vi "QuadRotor_Monitoring_LV4.vi"() -> ()   [LabVIEW 2015]
uses:
  <vilib>/Instr/_visa.llb/VISA Set IO Buffer Mask.ctl
  <vilib>/Instr/_visa.llb/VISA Configure Serial Port (Instr).vi
panel:
  out "GPS_TRANSPORT_Distance":dbl(slide) scale=0.0..200.0
  out "GPS_Home_Distance":dbl(slide) scale=0.0..200.0
  out "GPS_Speed_Gaud":ext(knob) scale=0.0..100.0
  out "GPS_LON_TRANSPORT":ext format="%#.7f"
  out "GPS_LAT_TRANSPORT":ext format="%#.7f"
  out "GPS_LON_HOME":ext format="%#.7f"
  out "GPS_LAT_HOME":ext format="%#.7f"
  out "MotorBackRf":dbl(slide) scale=1000.0..2000.0
  out "MotorBackLf":dbl(slide) scale=1000.0..2000.0
  out "MotorFrontRf":dbl(slide) scale=1000.0..2000.0
  out "MotorFrontLf":dbl(slide) scale=1000.0..2000.0
  in  "LON_TRANSPORT":i32=1001113510
  in  "LAT_TRANSPORT":i32=200300620
  in  "LON_HOME":i32=1001110710
  in  "LAT_HOME":i32=200292880
  out "(GPS_numSat)":u16(slide) scale=0.0..20.0 scale format="%#_4g"
  out "return count 2":u32
  out "Roob":i32
  out "Altitude_(Auto)":ext format="%#_3g"
  in  "Set_ATL_(Auto)":dbl=12.0
  out "string":string
  out "Mode":ext format="%.2f"
  out "Altitude":dbl(slide) scale=0.0..20.0
  out "Altitude":ext format="%.2f"
  out "Yaw":dbl(knob) scale=-180.0..180.0
  out "Pitch":dbl(knob) scale=-90.0..90.0
  out "Roll":dbl(knob) scale=-90.0..90.0
  in  "Write to Quad":bool
  out "Header_58":u8
  out "GPS_LONGTITUDE":ext format="%#.7f"
  out "GPS_LATTITUDE":ext format="%#.7f"
  out "return count":u32
  in  "stop":bool
  in  "VISA Serial Data":refnum<visa-resource-name>
  # "Quad Rotor Monitoring and Control with GPS Waypoint"
  # "Data Write to Autonomous Quad Rotor (LAT 9 Point), (LON 10 Point) with Google Map tracking Navigator"
  # "Ex  13.8591411 = 138591411 , 100.5231704 = 1005231704 Using in integer  I32"
  # "GPS Status and Monitoring"
  # "Km/h"
  # "9 Point"
  # "10 Point"
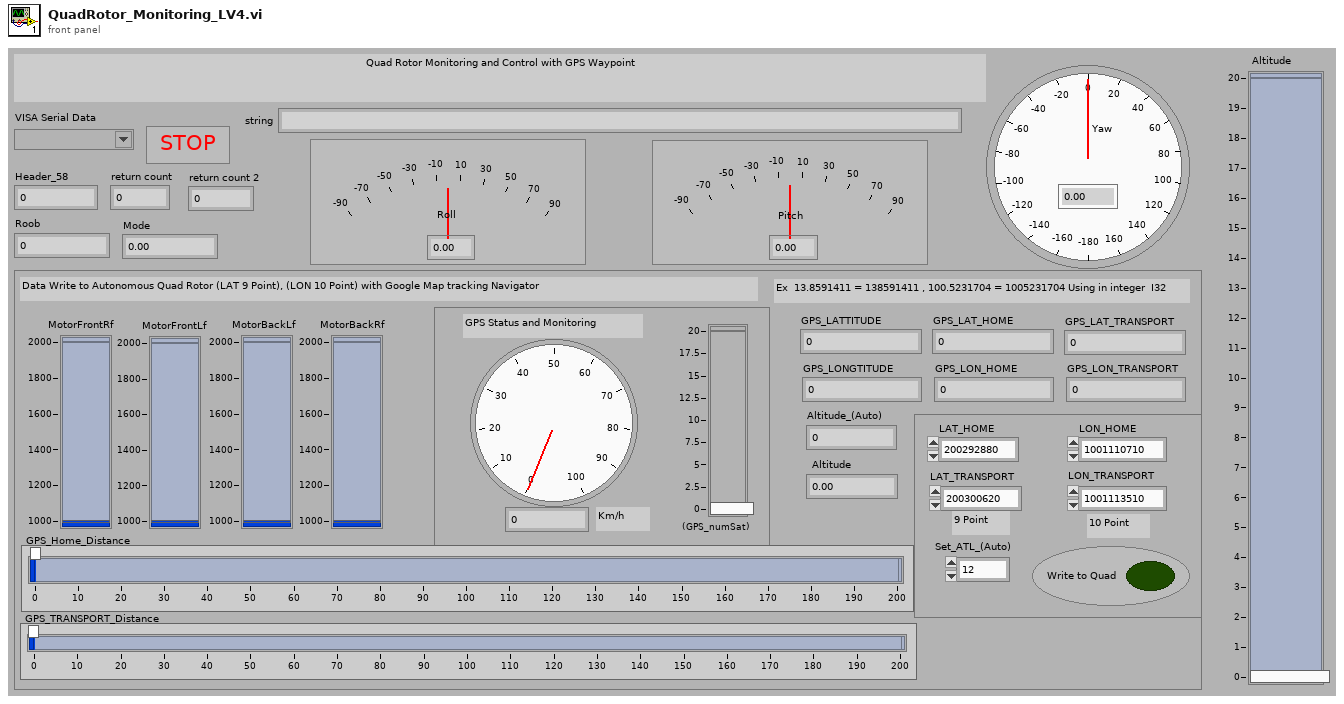
[diagram p1: front panel]
types:
  T1 = typedef "VISA Set IO Buffer Mask.ctl" = u16
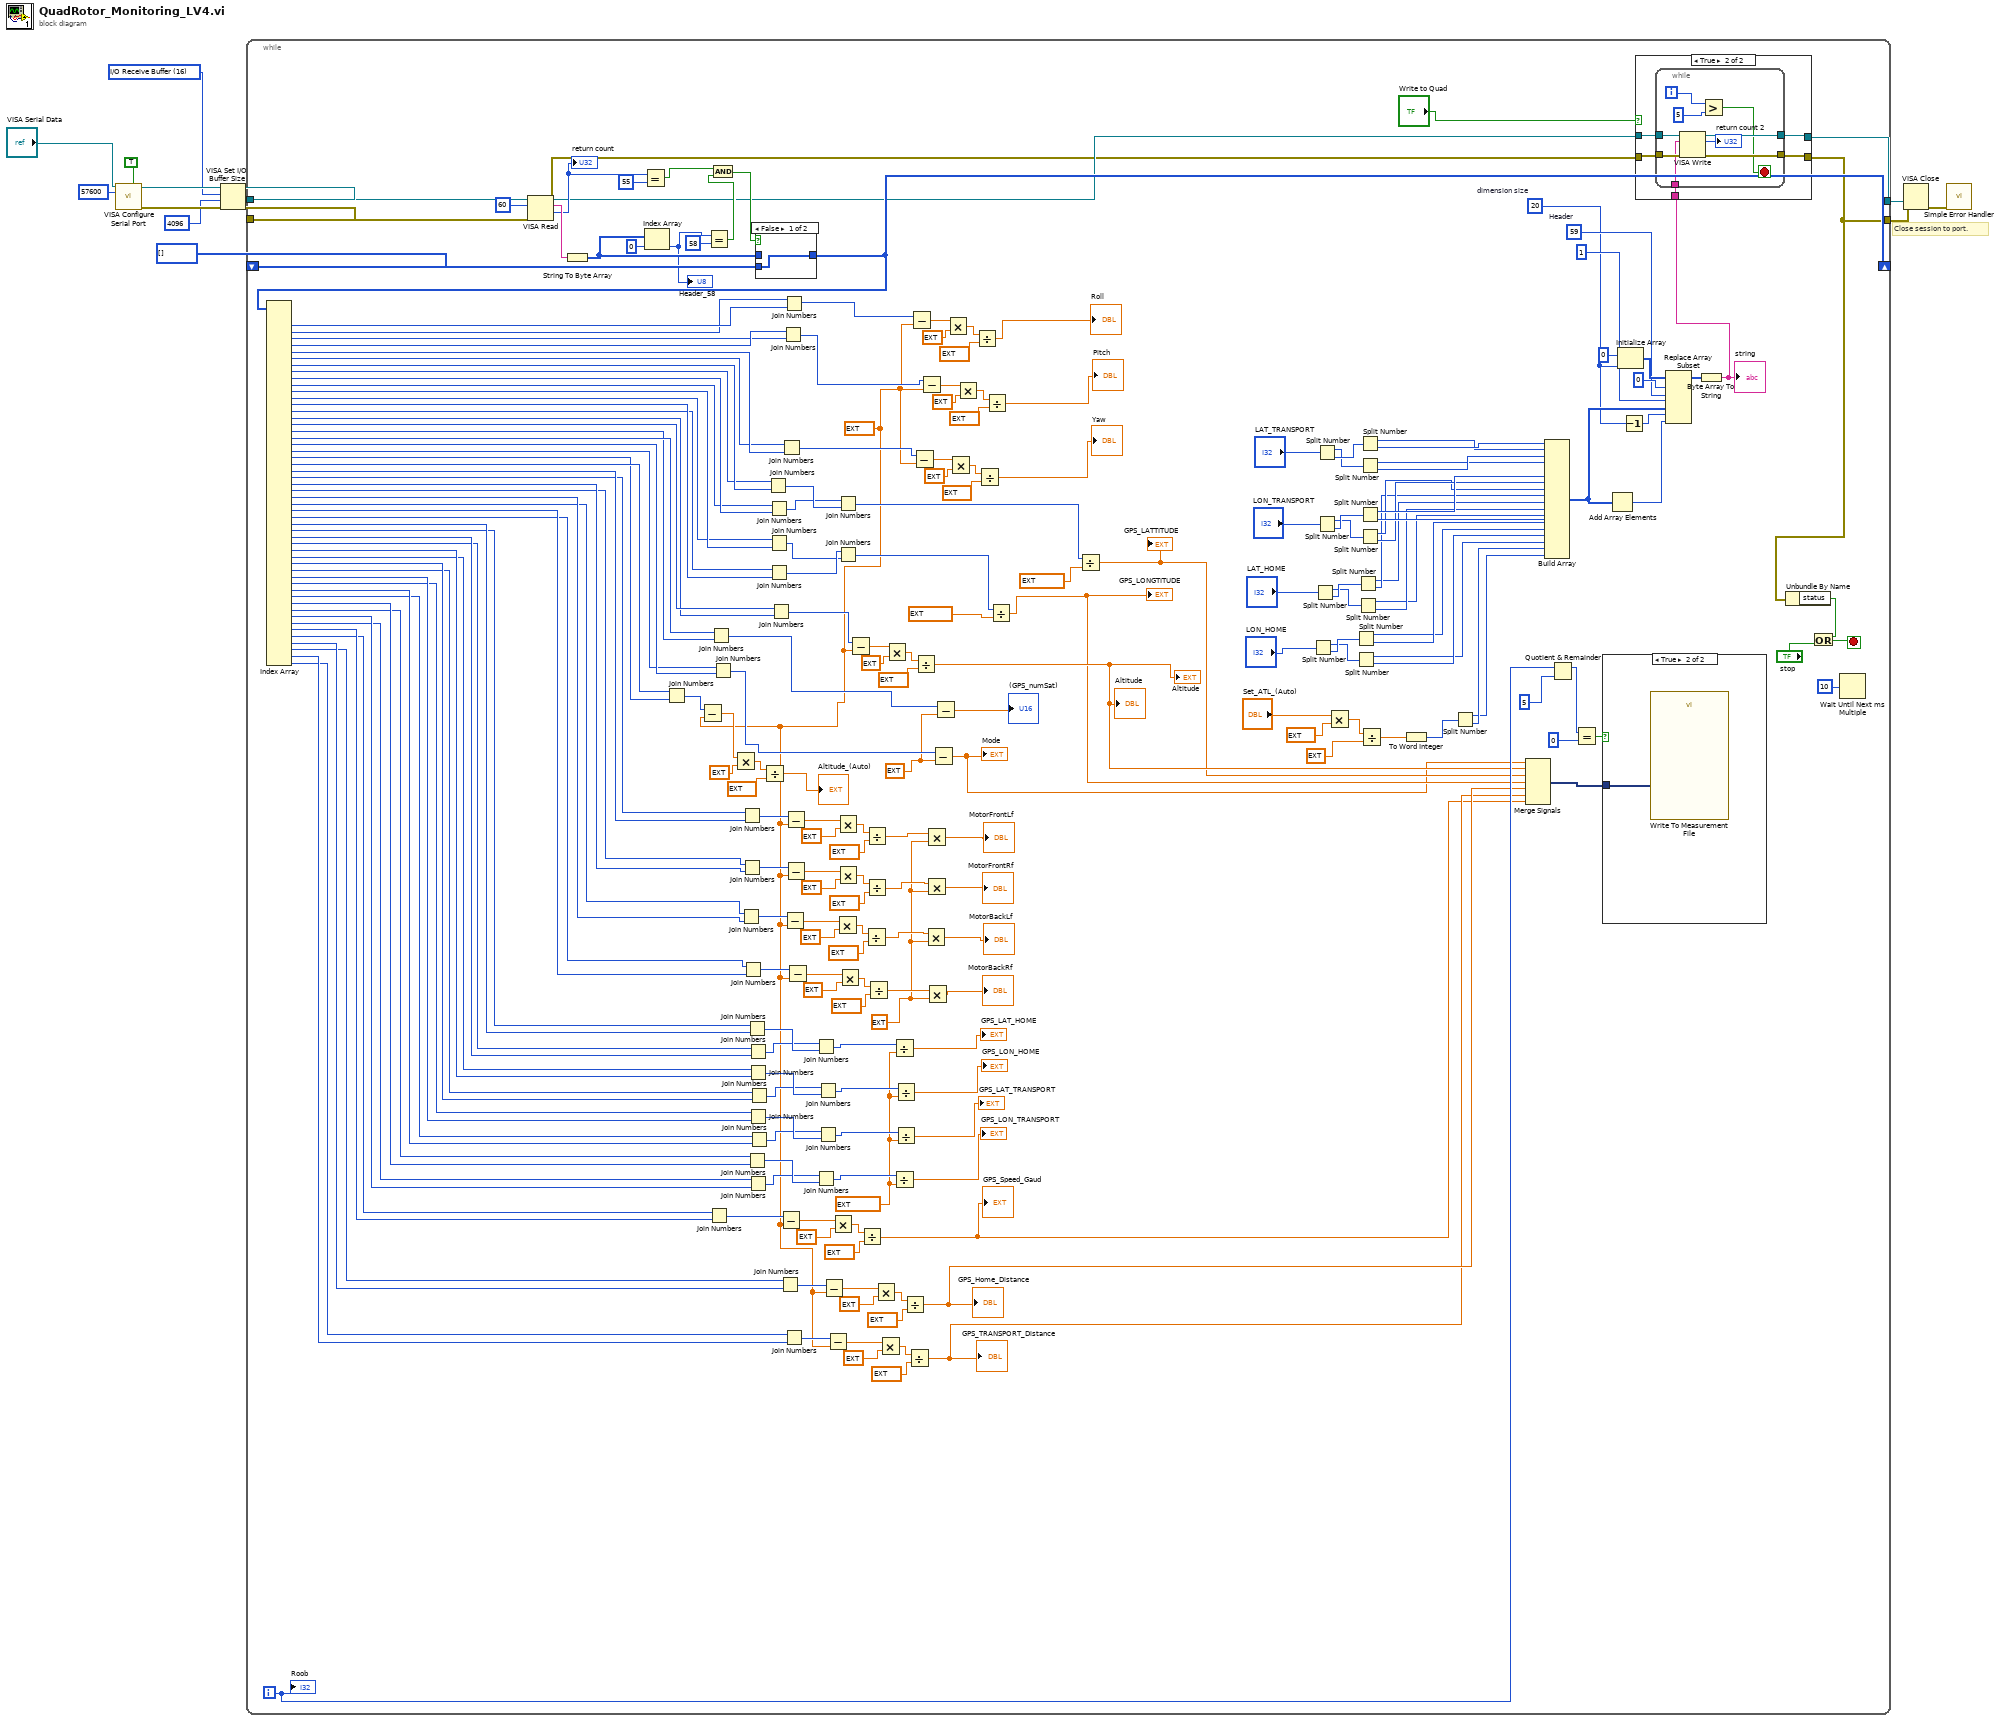
[diagram p0: block diagram]
diagram:
  w10 = T1 16 items=["I/O Receive Buffer"=16, "I/O Transmit Buffer"=32, "I/O Receive and Transmit Buffer"=48] ("Mask")
  # "Close session to port."
  n1 = call-poly "VISA Configure Serial Port"("VISA resource name"="VISA Serial Data", "Enable Termination\nChar (T)"=TRUE ("Enable Termination\nChar (T)"), "baud rate (9600)"=u32 57600) -> ("VISA resource name out"=w12:refnum<visa-resource-name>, "error out"=w11:errorcluster)  [unwired: 7 in, 4 out]
  n2 = VISA Set I/O Buffer Size(VISA resource name=w12, mask (16)=w10, size (4096)=u32 4096, error in (no error)=w11) -> (VISA resource name out=w8:refnum<visa-resource-name>, error out=w6:errorcluster)
  n3 = while {
    tunnel: [w208] -> w7
    tunnel: w8 -> [w249]
    tunnel: [w207] -> w5
    tunnel: w6 -> [w248]
    shift-right: [w218] -> _
    shift-left: u8[] [] ("unsigned byte array") -> [w219]
    i -> [w118]
    stop <- w252 stop-if-true
    w59 = ext 10000000.0 ("y")
    w78 = ext 10.0 ("y")
    w129 = 20  # dimension size
    w176 = u8 59  # Header
    w122 = ext 255.0 ("y")
    w25 = ext 32767.0 ("y")
    n4 = VISA Read(VISA resource name=w249, byte count=u32 60, error in (no error)=w248) -> (VISA resource name out=w210:refnum<visa-resource-name>, read buffer=w222:string, return count=w215:u32, error out=w209:errorcluster)
    "return count" <- w215
    n5 = String To Byte Array(string=w222) -> (unsigned byte array=w220:u8[])
    n6 = Equal?(x=w215, y=u32 55) -> (x = y?=w213:bool)
    n7 = Index Array(array=w220, index=0) -> (element=w212:u8)
    "Header_58" <- w212
    n8 = Equal?(x=w212, y=u8 58) -> (x = y?=w217:bool)
    n9 = And(x=w213, y=w217) -> (x .and. y?=w216:bool)
    n10 = case shown="False" w216 {
      tunnel: w220 -> [_ w271]
      tunnel: [w270 w271] -> w218
      tunnel: w219 -> [w270 _]
      frame False {
      }
      frame True {
      }
    }
    n11 = Index Array(array=w218) -> (element #2=w242:u8, element #3=w241:u8, element #4=w239:u8, element #5=w240:u8, element #6=w246:u8, element #7=w245:u8, element #8=w244:u8, element #9=w243:u8, element #10=w203:u8, element #11=w202:u8, element #12=w199:u8, element #13=w198:u8, element #14=w197:u8, element #15=w196:u8, element #16=w187:u8, element #17=w193:u8, element #18=w185:u8, element #19=w186:u8, element #20=w184:u8, element #21=w183:u8, element #22=w140:u8, element #23=w141:u8, element #24=w94:u8, element #25=w93:u8, element #26=w92:u8, element #27=w91:u8, element #28=w90:u8, element #29=w89:u8, element #30=w88:u8, element #31=w87:u8, element #32=w53:u8, element #33=w52:u8, element #34=w51:u8, element #35=w50:u8, element #36=w49:u8, element #37=w48:u8, element #38=w47:u8, element #39=w46:u8, element #40=w45:u8, element #41=w44:u8, element #42=w43:u8, element #43=w42:u8, element #44=w41:u8, element #45=w40:u8, element #46=w39:u8, element #47=w38:u8, element #48=w37:u8, element #49=w36:u8, element #50=w24:u8, element #51=w23:u8, element #52=w22:u8, element #53=w21:u8)  [unwired: 53 in, 1 out]
    n12 = Join Numbers(hi=w141, lo=w140) -> ((hi.lo)=w139:u16)
    n13 = Subtract(x=w139, y=w25) -> (x-y=w135:ext)
    n14 = Join Numbers(hi=w36, lo=w37) -> ((hi.lo)=w54:u16)
    n15 = Join Numbers(hi=w186, lo=w185) -> ((hi.lo)=w121:u16)
    n16 = Join Numbers(hi=w183, lo=w184) -> ((hi.lo)=w124:u16)
    n17 = Multiply(x=w135, y=ext 100.0) -> (x*y=w137:ext)
    n18 = Join Numbers(hi=w89, lo=w90) -> ((hi.lo)=w100:u16)
    n19 = Join Numbers(hi=w93, lo=w94) -> ((hi.lo)=w110:u16)
    n20 = Join Numbers(hi=w91, lo=w92) -> ((hi.lo)=w105:u16)
    n21 = Join Numbers(hi=w87, lo=w88) -> ((hi.lo)=w95:u16)
    n22 = Join Numbers(hi=w52, lo=w53) -> ((hi.lo)=w75:u16)
    n23 = Join Numbers(hi=w40, lo=w41) -> ((hi.lo)=w66:u16)
    n24 = Join Numbers(hi=w50, lo=w51) -> ((hi.lo)=w74:u16)
    n25 = Join Numbers(hi=w38, lo=w39) -> ((hi.lo)=w65:u16)
    n26 = Join Numbers(hi=w48, lo=w49) -> ((hi.lo)=w72:u16)
    n27 = Join Numbers(hi=w44, lo=w45) -> ((hi.lo)=w69:u16)
    n28 = Join Numbers(hi=w46, lo=w47) -> ((hi.lo)=w71:u16)
    n29 = Join Numbers(hi=w42, lo=w43) -> ((hi.lo)=w68:u16)
    n30 = Divide(x=w137, y=ext 32767.0) -> (x/y=→"Altitude_(Auto)":ext)
    n31 = Join Numbers(hi=w243, lo=w244) -> ((hi.lo)=w201:u16)
    n32 = Join Numbers(hi=w202, lo=w203) -> ((hi.lo)=w200:u16)
    n33 = Join Numbers(hi=w198, lo=w199) -> ((hi.lo)=w181:u16)
    n34 = Join Numbers(hi=w196, lo=w197) -> ((hi.lo)=w182:u16)
    n35 = Join Numbers(hi=w193, lo=w187) -> ((hi.lo)=w188:u16)
    n36 = Join Numbers(hi=w23, lo=w24) -> ((hi.lo)=w31:u16)
    n37 = Subtract(x=w54, y=w25) -> (x-y=w57:ext)
    n38 = Join Numbers(hi=w245, lo=w246) -> ((hi.lo)=w228:u16)
    n39 = Join Numbers(hi=w240, lo=w239) -> ((hi.lo)=w223:u16)
    n40 = Join Numbers(hi=w241, lo=w242) -> ((hi.lo)=w237:u16)
    n41 = Join Numbers(hi=w21, lo=w22) -> ((hi.lo)=w26:u16)
    n42 = Subtract(x=w100, y=w25) -> (x-y=w103:ext)
    n43 = Subtract(x=w110, y=w25) -> (x-y=w113:ext)
    n44 = Subtract(x=w105, y=w25) -> (x-y=w108:ext)
    n45 = Subtract(x=w95, y=w25) -> (x-y=w98:ext)
    n46 = Join Numbers(hi=w74, lo=w75) -> ((hi.lo)=w73:u32)
    n47 = Join Numbers(hi=w65, lo=w66) -> ((hi.lo)=w64:u32)
    n48 = Join Numbers(hi=w71, lo=w72) -> ((hi.lo)=w70:u32)
    n49 = Join Numbers(hi=w68, lo=w69) -> ((hi.lo)=w67:u32)
    n50 = Subtract(x=w31, y=w25) -> (x-y=w34:ext)
    n51 = Subtract(x=w26, y=w25) -> (x-y=w29:ext)
    n52 = Multiply(x=w57, y=ext 100.0) -> (x*y=w58:ext)
    n53 = Multiply(x=w103, y=ext 185.0) -> (x*y=w104:ext)
    n54 = Join Numbers(hi=w200, lo=w201) -> ((hi.lo)=w205:u32)
    n55 = Join Numbers(hi=w182, lo=w181) -> ((hi.lo)=w195:u32)
    n56 = Multiply(x=w113, y=ext 185.0) -> (x*y=w114:ext)
    n57 = Multiply(x=w108, y=ext 185.0) -> (x*y=w109:ext)
    n58 = Multiply(x=w98, y=ext 185.0) -> (x*y=w99:ext)
    n59 = Subtract(x=w188, y=w25) -> (x-y=w192:ext)
    n60 = Divide(x=w58, y=ext 32767.0) -> (x/y=w15:ext)
    "GPS_Speed_Gaud" <- w15
    n61 = Divide(x=w104, y=ext 32767.0) -> (x/y=w81:ext)
    n62 = Divide(x=w114, y=ext 32767.0) -> (x/y=w79:ext)
    n63 = Divide(x=w109, y=ext 32767.0) -> (x/y=w80:ext)
    n64 = Divide(x=w99, y=ext 32767.0) -> (x/y=w86:ext)
    n65 = Multiply(x=w34, y=ext 200.0) -> (x*y=w35:ext)
    n66 = Multiply(x=w29, y=ext 200.0) -> (x*y=w30:ext)
    n67 = Multiply(x=w192, y=ext 100.0) -> (x*y=w190:ext)
    n68 = Divide(x=w73, y=w59) -> (x/y=→"GPS_LAT_HOME":ext)
    n69 = Divide(x=w64, y=w59) -> (x/y=→"GPS_LON_TRANSPORT":ext)
    n70 = Divide(x=w70, y=w59) -> (x/y=→"GPS_LON_HOME":ext)
    n71 = Divide(x=w67, y=w59) -> (x/y=→"GPS_LAT_TRANSPORT":ext)
    n72 = Divide(x=w35, y=ext 32767.0) -> (x/y=w17:ext)
    "GPS_Home_Distance" <- w17
    n73 = Divide(x=w30, y=ext 32767.0) -> (x/y=w16:ext)
    "GPS_TRANSPORT_Distance" <- w16
    n74 = Subtract(x=w237, y=w25) -> (x-y=w236:ext)
    n75 = Subtract(x=w228, y=w25) -> (x-y=w232:ext)
    n76 = Divide(x=w190, y=ext 32767.0) -> (x/y=w20:ext)
    "Altitude" <- w20
    "Altitude" <- w20
    n77 = Subtract(x=w223, y=w25) -> (x-y=w227:ext)
    n78 = Multiply(x=w81, y=w78) -> (x*y=→"MotorBackLf":ext)
    n79 = Multiply(x=w79, y=w78) -> (x*y=→"MotorFrontLf":ext)
    n80 = Multiply(x=w80, y=w78) -> (x*y=→"MotorFrontRf":ext)
    n81 = Multiply(x=w86, y=w78) -> (x*y=→"MotorBackRf":ext)
    n82 = Subtract(x=w124, y=w122) -> (x-y=w14:ext)
    "Mode" <- w14
    n83 = Subtract(x=w121, y=w122) -> (x-y=→"(GPS_numSat)":ext)
    n84 = Multiply(x=w236, y=ext 180.0) -> (x*y=w234:ext)
    n85 = Multiply(x=w232, y=ext 180.0) -> (x*y=w230:ext)
    n86 = Multiply(x=w227, y=ext 180.0) -> (x*y=w225:ext)
    n87 = Divide(x=w234, y=ext 32767.0) -> (x/y=→"Roll":ext)
    n88 = Divide(x=w230, y=ext 32767.0) -> (x/y=→"Yaw":ext)
    n89 = Divide(x=w225, y=ext 32767.0) -> (x/y=→"Pitch":ext)
    n90 = Divide(x=w195, y=ext 10000000.0) -> (x/y=w18:ext)
    "GPS_LONGTITUDE" <- w18
    n91 = Divide(x=w205, y=ext 10000000.0) -> (x/y=w19:ext)
    "GPS_LATTITUDE" <- w19
    n92 = Split Number(x="LON_HOME") -> (hi(x)=w169:u16, lo(x)=w170:u16)
    n93 = Split Number(x="LAT_HOME") -> (hi(x)=w171:u16, lo(x)=w172:u16)
    n94 = Split Number(x="LON_TRANSPORT") -> (hi(x)=w173:u16, lo(x)=w174:u16)
    n95 = Split Number(x="LAT_TRANSPORT") -> (hi(x)=w151:u16, lo(x)=w152:u16)
    n96 = Multiply(x="Set_ATL_(Auto)", y=ext 32767.0) -> (x*y=w144:ext)
    n97 = Split Number(x=w170) -> (hi(x)=w155:u8, lo(x)=w156:u8)
    n98 = Split Number(x=w169) -> (hi(x)=w153:u8, lo(x)=w154:u8)
    n99 = Split Number(x=w172) -> (hi(x)=w159:u8, lo(x)=w160:u8)
    n100 = Split Number(x=w171) -> (hi(x)=w157:u8, lo(x)=w158:u8)
    n101 = Split Number(x=w174) -> (hi(x)=w163:u8, lo(x)=w164:u8)
    n102 = Split Number(x=w173) -> (hi(x)=w161:u8, lo(x)=w162:u8)
    n103 = Split Number(x=w152) -> (hi(x)=w167:u8, lo(x)=w168:u8)
    n104 = Split Number(x=w151) -> (hi(x)=w165:u8, lo(x)=w166:u8)
    n105 = Divide(x=w144, y=ext 100.0) -> (x/y=w142:ext)
    n106 = To Word Integer(number=w142) -> (16bit integer=w145:i16)
    n107 = Split Number(x=w145) -> (hi(x)=w146:u8, lo(x)=w147:u8)
    n108 = Merge Signals(w14, w20, w19, w18, w17, w16, w15) -> (w120:dynamicdata)
    n109 = Build Array(w168, w167, w166, w165, w164, w163, w162, w161, w160, w159, w158, w157, w156, w155, w154, w153, w147, w146) -> (w132:u8[])
    n110 = Quotient & Remainder(x=w118, y=u32 5) -> (x-y*floor(x/y)=w115:u32)  [unwired: 1 out]
    n111 = Equal?(x=w115, y=u32 0) -> (x = y?=w117:bool)
    n112 = case shown="True" w117 {
      tunnel: w120 -> [_ w253]
      frame False {
      }
      frame True {
        n113 = call "Write To Measurement File"("Signals"=w253) -> ()  [unwired: 16 in, 3 out]
      }
    }
    n114 = Add Array Elements(numeric array=w132) -> (sum=w131:u8)
    n115 = Initialize Array(u8 0, w129) -> (w180:u8[])
    n116 = Decrement(x=w129) -> (x-1=w130:i32)
    n117 = Replace Array Subset(array=w180, new element #1=w176, index #1=0 ("index"), new element #2=w132, index #2=1 ("index"), new element #3=w131, index #3=w130) -> (w175:u8[])
    n118 = Byte Array To String(unsigned byte array=w175) -> (string=w150:string)
    "string" <- w150
    n119 = case shown="True" "Write to Quad" {
      tunnel: w210 -> [w254 w260]
      tunnel: w209 -> [w255 w257]
      tunnel: [w254 w259] -> w208
      tunnel: [w255 w258] -> w207
      tunnel: w150 -> [_ w256]
      frame False {
      }
      frame True {
        n120 = while {
          tunnel: w260 -> [w269]
          tunnel: [w268] -> w259
          tunnel: [w267] -> w258
          tunnel: w257 -> [w266]
          tunnel: w256 -> [w265]
          i -> [w263]
          stop <- w261 stop-if-true
          n121 = VISA Write(VISA resource name=w269, write buffer=w265, error in (no error)=w266) -> (VISA resource name out=w268:refnum<visa-resource-name>, return count=→"return count 2":u32, error out=w267:errorcluster)
          n122 = Greater?(x=w263, y=5) -> (0:w261:bool)
        }
      }
    }
    n123 = Unbundle By Name(w207) -> ("status"=w250:bool)
    n124 = Or(x=w250, y="stop") -> (x .or. y?=w252:bool)
    n125 = Wait Until Next ms Multiple(millisecond multiple=u32 10) -> ()  [unwired: 1 out]
    "Roob" <- w118
  }
  n126 = VISA Close(VISA resource name=w7, error in (no error)=w5) -> (error out=w9:errorcluster)
  n127 = call <vilib>:"Simple Error Handler.vi"("error in (no error)"=w9) -> ()  [unwired: 1 in, 8 out]
